vi "Read CAN Setting Value.vi"(8 "error in (no error)":errorcluster, 11 "Instrument Parameter":string[][](array[string])) -> (0 "error out":errorcluster, 2 "Output Cluster":T2={"CAN Cluster"=":memory:", "Select Interface"="CAN1", "Interface Baud Rate"=125000, "Data"=[]} {"Data"."CAN frame"."payload" format="%x"; "Data"."CAN frame"."timestamp" format="%<%.7X\n%x>T"; "Data"."CAN frame"."type" items=["CAN Data"=0, "CAN Remote"=1, "CAN Bus Error"=2, "CAN 2.0 Data"=8, "CAN FD Data"=16, "CAN FD+BRS Data"=24, "J1939 Data"=192, "Delay"=224, "Log Trigger"=225, "Start Trigger"=226]; "Data"."CAN frame"."identifier" format="%x"}, 3 "Input Cluster":T1)   [LabVIEW 2021, in "CAN.lvlib"]
uses:
  Output Parameter.ctl
  CAN Frame.ctl
  <vilib>/xnet/xnet.llb/XNET Frame Type CAN.ctl
  Input Parameter.ctl
  CAN.lvlib
  User Interface/User Interface.lvlib
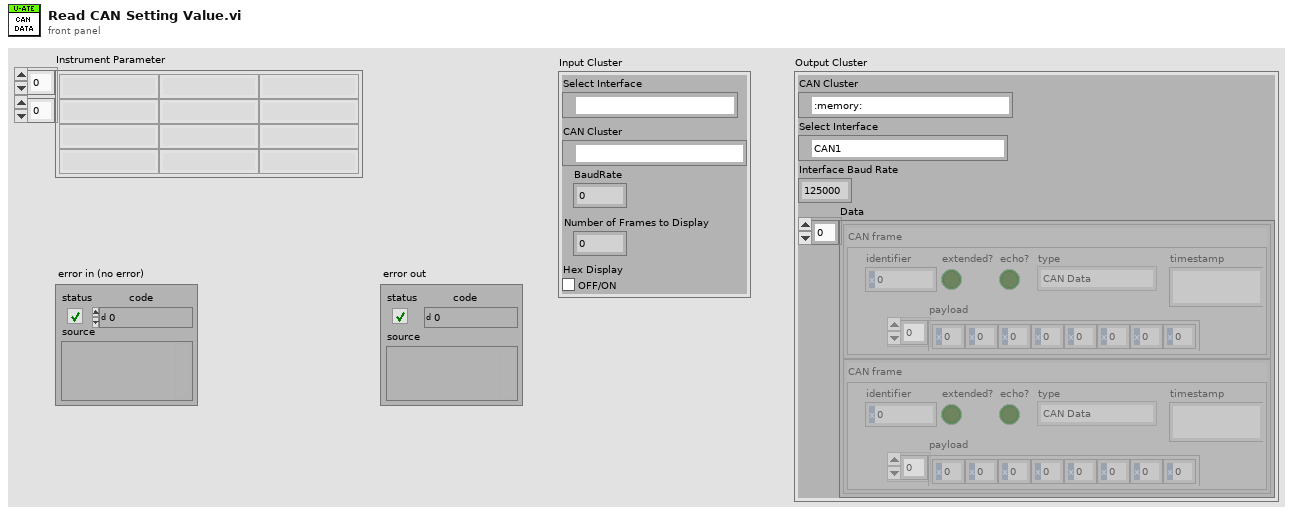
[diagram p1: front panel]
types:
  T1 = typedef "CAN.lvlib/Input Parameter.ctl" = cluster{"CAN Cluster":refnum<k21>, "Select Interface":refnum<k21>, "BaudRate":u32, "Number of Frames to Display":i32, "Hex Display":bool}
  T2 = typedef "CAN.lvlib/Output Parameter.ctl" = cluster{"CAN Cluster":refnum<k21>, "Select Interface":refnum<k21>, "Interface Baud Rate":u32, "Data":T3[]}
  T3 = typedef "CAN.lvlib/CAN Frame.ctl" = cluster{"CAN frame":cluster{"timestamp":timestamp, "payload":u8[], "identifier":u32, "type":T4, "extended?":bool, "echo?":bool}}
  T4 = typedef "XNET Frame Type CAN.ctl" = u8
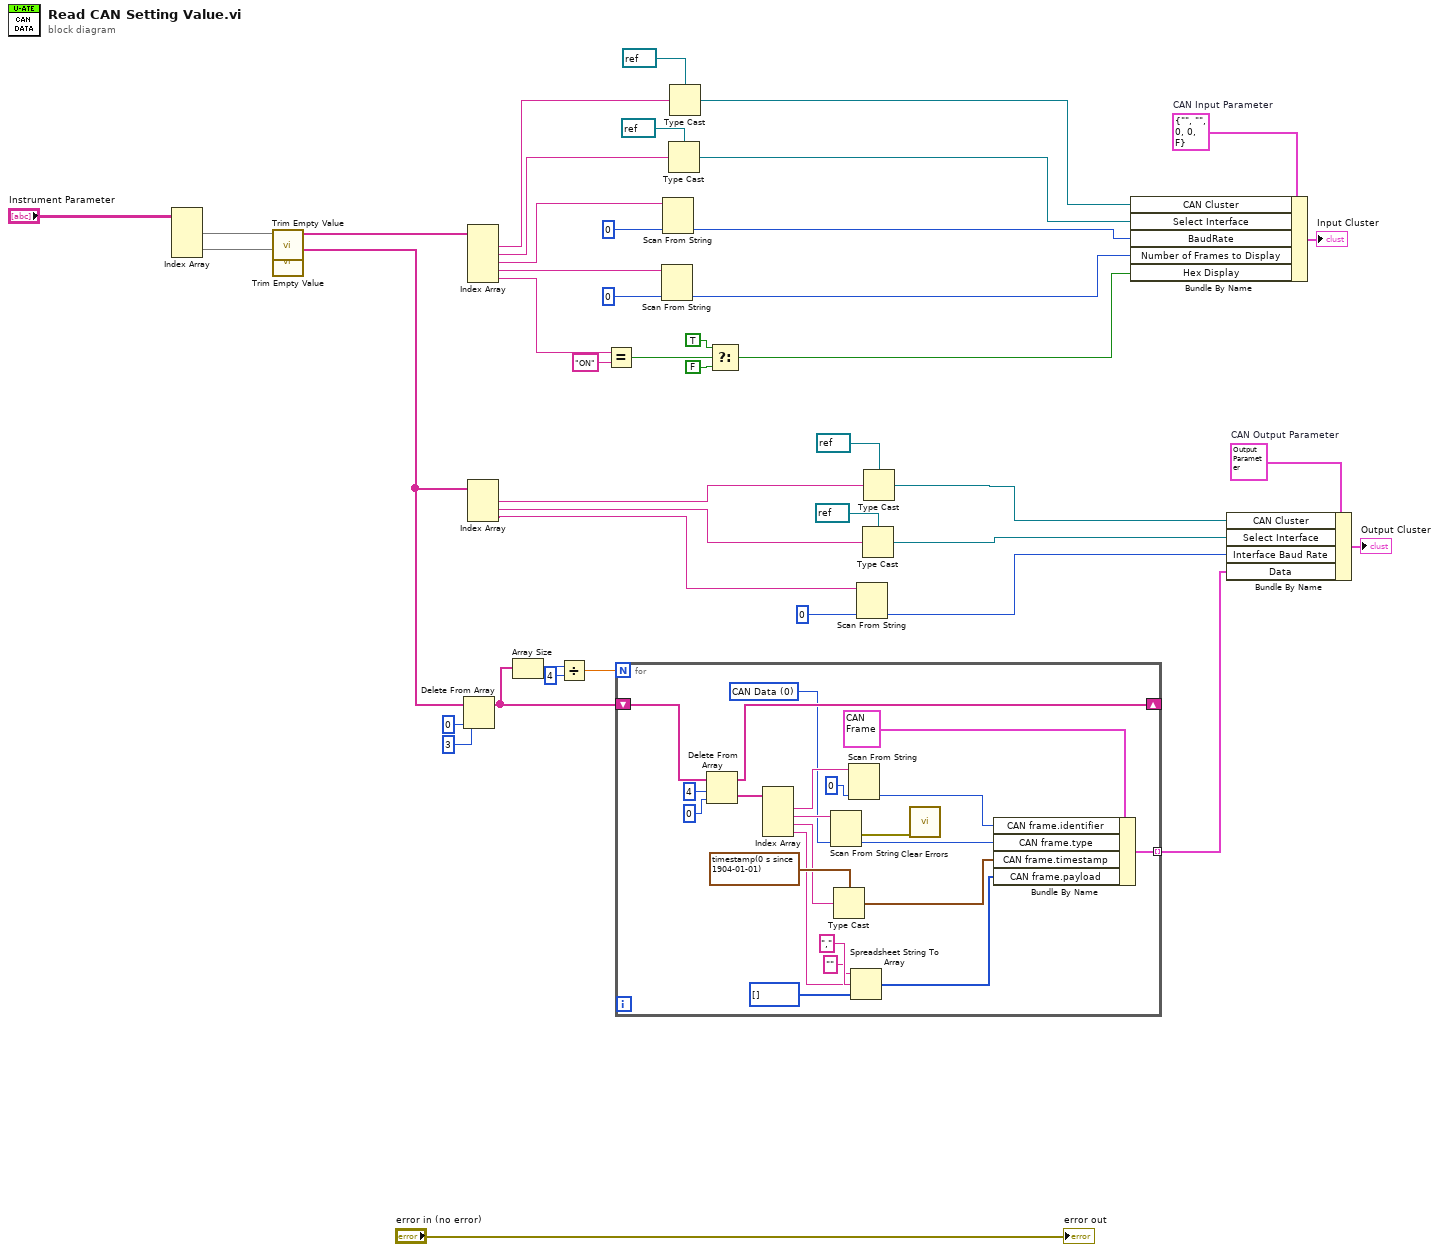
[diagram p0: block diagram]
diagram:
  w20 = T2 {"CAN Cluster"=":memory:", "Select Interface"="CAN1", "Interface Baud Rate"=125000, "Data"=[{"CAN frame"={"timestamp"=timestamp(0 s since 1904-01-01), "payload"=[], "identifier"=0, "type"=0, "extended?"=FALSE, "echo?"=FALSE}}, {"CAN frame"={"timestamp"=timestamp(0 s since 1904-01-01), "payload"=[], "identifier"=0, "type"=0, "extended?"=FALSE, "echo?"=FALSE}}]}  # CAN Output Parameter
  w39 = T1 {"CAN Cluster"="", "Select Interface"="", "BaudRate"=0, "Number of Frames to Display"=0, "Hex Display"=FALSE}  # CAN Input Parameter
  n1 = Index Array(array="Instrument Parameter") -> (element #1=w42:string[], element #2=w41:string[])  [unwired: 4 in]
  n2 = call "Trim Empty Value.vi"("Data In"=w42) -> ("Data Out"=w40:string[])  [unwired: 10 in]
  n3 = call "Trim Empty Value.vi"("Data In"=w41) -> ("Data Out"=w10:string[])  [unwired: 10 in]
  n4 = Delete From Array(array=w10, length=3, index=0) -> (array with subset deleted=w7:string[])  [unwired: 1 out]
  n5 = Index Array(array=w40) -> (element #1=w38:string, element #2=w37:string, element #3=w26:string, element #4=w23:string, element #5=w35:string)  [unwired: 5 in]
  n6 = Index Array(array=w10) -> (element #1=w16:string, element #2=w15:string, element #3=w14:string)  [unwired: 3 in]
  n7 = Array Size(array=w7) -> (size(s)=w6:i32)
  n8 = Divide(x=w6, y=4) -> (x/y=w4:dbl)
  n9 = Equal?(x=w35, y="ON") -> (x = y?=w33:bool)
  n10 = for {
    N: w4 -> [_]
    shift-right: [w63] -> _
    shift-left: w7 -> [w66]
    tunnel: [w47] -> w3 mode=indexing
    w45 = T4 0 items=["CAN Data"=0, "CAN Remote"=1, "CAN Bus Error"=2, "CAN 2.0 Data"=8, "CAN FD Data"=16, "CAN FD+BRS Data"=24, "J1939 Data"=192, "Delay"=224, "Log Trigger"=225, "Start Trigger"=226] ("CAN frame.type")
    n11 = Delete From Array(array=w66, length=4, index=0) -> (deleted portion=w62:string[], array with subset deleted=w63:string[])
    n12 = Index Array(array=w62) -> (element #1=w60:string, element #2=w57:string, element #3=w54:string, element #4=w49:string)  [unwired: 4 in]
    n13 = Scan From String(input string=w57, default 1=w45) -> (error out=w46:errorcluster, output 1=w56:T4)  [unwired: 3 in, 2 out]
    n14 = Type Cast(type=timestamp(0 s since 1904-01-01) ("CAN frame.timestamp"), x=w54) -> (*(type *) &x=w53:timestamp)
    n15 = Scan From String(input string=w60, default 1=u32 0 ("CAN frame.identifier")) -> (output 1=w58:u32)  [unwired: 3 in, 3 out]
    n16 = Spreadsheet String To Array(delimiter (Tab)=",", format string="", spreadsheet string=w49, array type (2D Dbl)=u8[] [] ("CAN frame.payload")) -> (array=w48:u8[])
    n17 = call <vilib>:"Clear Errors.vi"("error in (no error)"=w46) -> ()  [unwired: 5 in, 2 out]
    n18 = Bundle By Name(cluster=T3 {"CAN frame"={"timestamp"=timestamp(0 s since 1904-01-01), "payload"=[], "identifier"=0, "type"=0, "extended?"=FALSE, "echo?"=FALSE}}, "CAN frame.identifier"=w58, "CAN frame.type"=w56, "CAN frame.timestamp"=w53, "CAN frame.payload"=w48) -> (w47:T3)
  }
  n19 = Scan From String(input string=w23, default 1=0 ("Number of Frames to Display")) -> (output 1=w21:i32)  [unwired: 3 in, 3 out]
  n20 = Scan From String(input string=w26, default 1=u32 0 ("BaudRate")) -> (output 1=w24:u32)  [unwired: 3 in, 3 out]
  n21 = Type Cast(type=refnum<k21> refnum ("Select Interface"), x=w37) -> (*(type *) &x=w27:refnum<k21>)
  n22 = Type Cast(type=refnum<k21> refnum ("CAN Cluster"), x=w38) -> (*(type *) &x=w29:refnum<k21>)
  n23 = Select(t=TRUE, s=w33, f=FALSE) -> (s? t:f=w31:bool)
  n24 = Scan From String(input string=w14, default 1=u32 0 ("BaudRate")) -> (output 1=w11:u32)  [unwired: 3 in, 3 out]
  n25 = Type Cast(type=refnum<k21> refnum ("Select Interface"), x=w15) -> (*(type *) &x=w12:refnum<k21>)
  n26 = Type Cast(type=refnum<k21> refnum ("CAN Cluster"), x=w16) -> (*(type *) &x=w13:refnum<k21>)
  n27 = Bundle By Name(cluster=w39, "CAN Cluster"=w29, "Select Interface"=w27, "BaudRate"=w24, "Number of Frames to Display"=w21, "Hex Display"=w31) -> (→"Input Cluster":T1)
  n28 = Bundle By Name(cluster=w20, "CAN Cluster"=w13, "Select Interface"=w12, "Interface Baud Rate"=w11, "Data"=w3) -> (→"Output Cluster":T2)
  "error out" <- "error in (no error)"
